vi "Load Test Stand.vi"(8 "Error In":errorcluster, 9 "Select Test Stand":T1, 10 "App Base Path":path, 11 "Test Stand.lvclass":refnum<class "Generic Test Stand.lvclass">) -> (0 "Error Out":errorcluster, 1 "Test Stand Name":string, 3 "Specific Test Stand.lvclass":refnum<class "Generic Test Stand.lvclass">)   [LabVIEW 2019, in "TS Framework.lvlib"]
uses:
  TS Framework.lvlib
  Test Stand Names.ctl
  Generic Test Stand/Generic Test Stand.lvclass
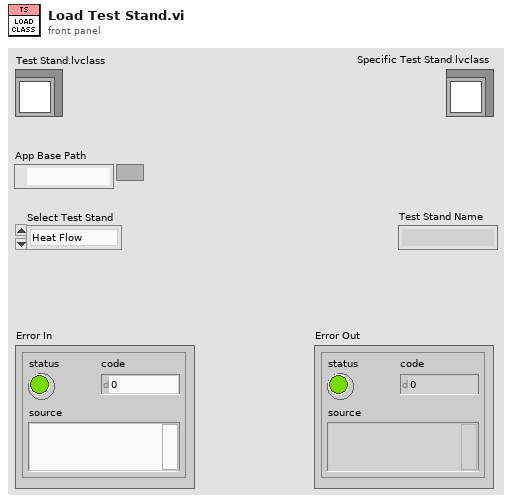
[diagram p1: front panel]
types:
  T1 = typedef "TS Framework.lvlib/Test Stand Names.ctl" = enum16{"Heat Flow", "LNG Boiling", "HTS", "Water Tunnel", "DeepU", "Cryo Sep"}
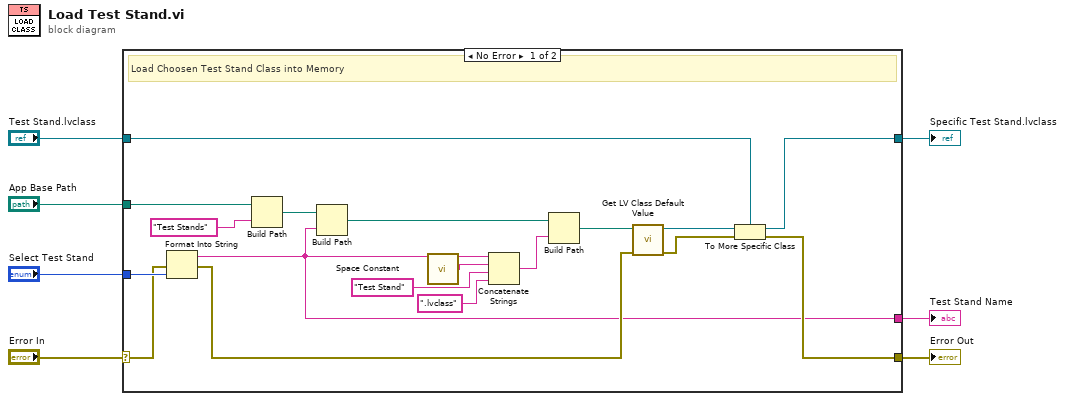
[diagram p0: block diagram]
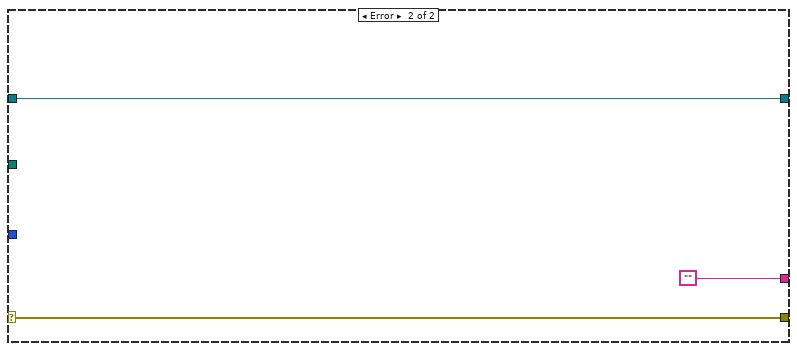
[diagram p2: hidden frame]
diagram:
  n1 = case shown="No Error" "Error In" {
    selector: "Error In" -> [w10 w28]
    tunnel: [w15 w28] -> w6
    tunnel: "Select Test Stand" -> [w25 _]
    tunnel: "Test Stand.lvclass" -> [w17 w27]
    tunnel: [w16 w27] -> w3
    tunnel: "App Base Path" -> [w11 _]
    tunnel: [w8 ""] -> w1
    frame No Error {
      # "Load Choosen Test Stand Class into Memory"
      n2 = Format Into String(error in=w10, w25) -> (resulting string=w8:string, error out=w9:errorcluster)  [unwired: 2 in]
      n3 = Build Path(base path=w11, name or relative path="Test Stands") -> (appended path=w13:path)
      n4 = Build Path(base path=w13, name or relative path=w8) -> (appended path=w14:path)
      n5 = call <vilib>:"Space Constant.vi"() -> ("String"=w23:string)
      n6 = Concatenate Strings(w8, w23, "Test Stand" ("name or relative path"), ".lvclass" ("string")) -> (w22:string)
      n7 = Build Path(base path=w14, name or relative path=w22) -> (appended path=w20:path)
      n8 = call <vilib>:"Get LV Class Default Value.vi"("error in (no error)"=w9, "class path"=w20) -> ("error out"=w18:errorcluster, "object"=w19:refnum<class>)  [unwired: 8 in]
      n9 = To More Specific Class(target class=w17, reference=w19, error in=w18) -> (specific class reference=w16:refnum<class "Generic Test Stand.lvclass">, error out=w15:errorcluster)
    }
    frame Error {
    }
  }
  "Error Out" <- w6
  "Specific Test Stand.lvclass" <- w3
  "Test Stand Name" <- w1
